vi "GetSampleCalFilePath.vi"(8 "Error In":errorcluster, 11 "Position":i16) -> (0 "Error Out":errorcluster, 3 "path":path)   [LabVIEW 2019]
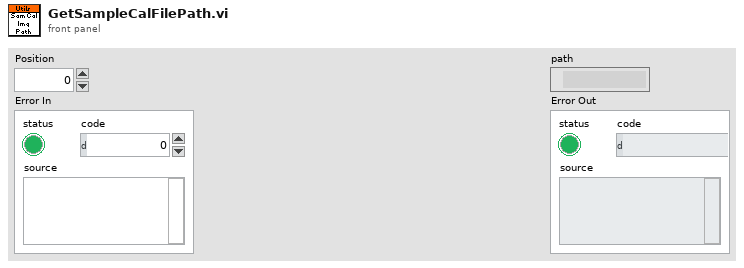
[diagram p1: front panel]
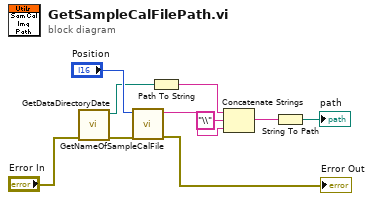
[diagram p0: block diagram]
diagram:
  n1 = call "GetDataDirectoryDate.vi"("Error In"="Error In") -> ("Error Out"=w10:errorcluster, "path"=w8:path)  [unwired: 9 in]
  n2 = call "GetNameOfSampleCalFile.vi"("Error In"=w10, "Position"="Position") -> ("Error Out"=→"Error Out":errorcluster, "Filename"=w5:string)  [unwired: 8 in]
  n3 = Path To String(path=w8) -> (string=w7:string)
  n4 = Concatenate Strings(w7, "\\" ("string"), w5) -> (w4:string)
  n5 = String To Path(string=w4) -> (path=→"path":path)
